vi "Save Front panel to Image.vi"(8 "error in (no error)":errorcluster, 9 "FileName":string, 10 "path include file name":path, 11 "vi reference":refnum<vi>) -> (0 "error out 2":errorcluster, 3 "path":path)   [LabVIEW 2021]
doc: "保存vi前面板为png图片。"
panel:
  in  "s":bool
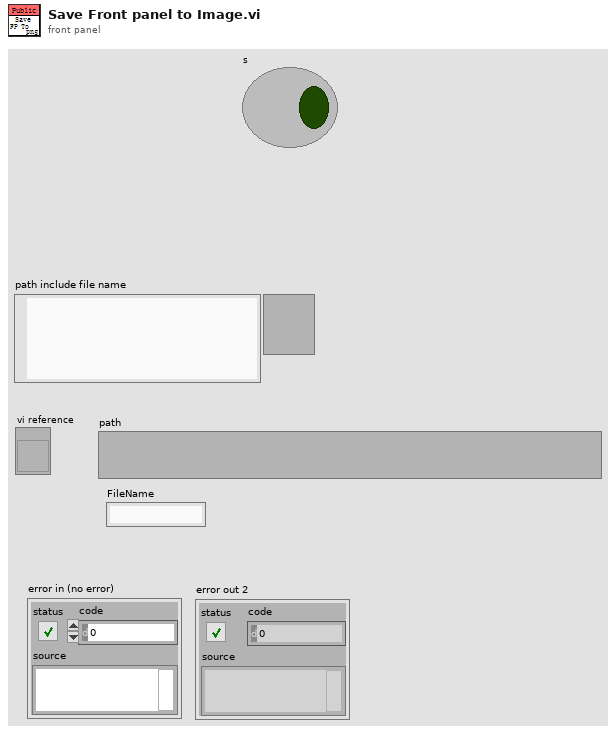
[diagram p1: front panel]
types:
  T1 = typedef "imagedata.ctl" = cluster{"image type":i32, "image depth":i32, "image":u8[], "mask":u8[], "colors":u32[], "Rectangle":cluster{"left":i16, "top":i16, "right":i16, "bottom":i16}}
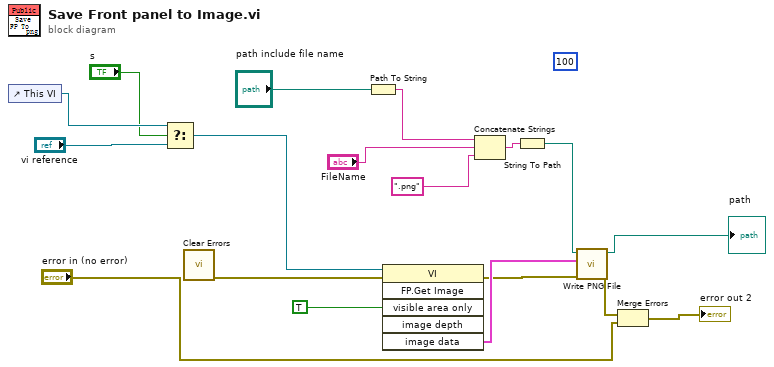
[diagram p0: block diagram]
diagram:
  (unwired) 100 ("quality (80)")
  n1 = control-ref of="This VI"() -> (w9:refnum<vi>)
  n2 = Select(t=w9, s="s", f="vi reference") -> (s? t:f=w10:refnum<vi>)
  n3 = call <vilib>:"Clear Errors.vi"() -> ("error out"=w3:errorcluster)  [unwired: 6 in, 1 out]
  n4 = Path To String(path="path include file name") -> (string=w7:string)
  n5 = invoke on="Invoke Node" class="VI" method="FP.Get Image"(reference=w10, error in=w3, "visible area only"=TRUE) -> (error out=w14:errorcluster, "image data"=w18:T1)  [unwired: 3 in, 4 out]
  n6 = Concatenate Strings(w7, "FileName", ".png" ("name or relative path")) -> (w12:string)
  n7 = String To Path(string=w12) -> (path=w6:path)
  n8 = call <vilib>:"Write PNG File.vi"("error in (no error)"=w14, "image data"=w18, "path to PNG file"=w6) -> ("error out"=w13:errorcluster, "path"=→"path":path)  [unwired: 7 in]
  n9 = Merge Errors(w13, "error in (no error)") -> (→"error out 2":errorcluster)
